vi "Lab Panel V4.83.vi"() -> ()   [LabVIEW 2013] (continued)
                  tunnel: w3955 -> [_ w3965]
                  frame False {
                  }
                  frame True {
                    n2340 = local read "TEMP START LAB03-1"() -> (w3971:cluster{"TL":dbl, "TN":dbl})
                    n2341 = local read "FAIL LAB03-1"() -> (w3962:cluster{"LO":dbl, "HI":dbl})
                    n2342 = local read "TDMS LAB03-1"() -> (w3970:refnum<k34>)
                    n2343 = local read "SET LAB03-1"() -> (w3967:T5)
                    n2344 = local read "DISP LAB03-1"() -> (w3968:T4)
                    n2345 = local read "SIG LAB03-1"() -> (w3972:T2)
                    n2346 = local read "RESULT LAB03-1"() -> (w3959:bool)
                    n2347 = Bundle("FAIL LAB03-1"=w3962, "SIG LAB03-1"=w3972, "TEMP START LAB03-1"=w3971, "DISP LAB03-1"=w3968, "SET LAB03-1"=w3967, "TDMS LAB03-1"=w3970) -> (w3957:T32)  [unwired: 1 in]
                    n2348 = call "sub vi - cycle&temp fail v6.vi"("Amps Lo?"=w3969, "Input Cluster"=w3957, "SELECT"=w3966, "Amps Hi?"=w3965, "Result In"=w3959) -> ("(FAIL) out"=w3961:cluster{"FAIL LO":dbl, "FAIL HI":dbl}, "(DISP) out"=w3964:T4, "T-RISE"=w3958:cluster{"T-RISE (L)":dbl, "T-RISE (N)":dbl}, "Result Out"=w3960:bool, "file error"=w3963:errorcluster)  [unwired: 10 in]
                    n2349 = local write "TEMP RISE LAB03-1"(w3958) -> ()
                    n2350 = local write "FAIL LAB03-1"(w3961) -> ()
                    n2351 = local write "DISP LAB03-1"(w3964) -> ()
                    n2352 = local write "RESULT LAB03-1"(w3960) -> ()
                    n2353 = local write "data file error"(w3963) -> ()
                  }
                }
              }
              frame #5 {
                # "LAB03-2"
                n2354 = case shown="True" w3974 {
                  tunnel: w3976 -> [_ w3989]
                  tunnel: w3973 -> [_ w3986]
                  tunnel: w3975 -> [_ w3985]
                  frame False {
                  }
                  frame True {
                    n2355 = local read "TEMP START LAB03-2"() -> (w3991:cluster{"TL":dbl, "TN":dbl})
                    n2356 = local read "FAIL LAB03-2"() -> (w3982:cluster{"LO":dbl, "HI":dbl})
                    n2357 = local read "TDMS LAB03-2"() -> (w3990:refnum<k34>)
                    n2358 = local read "SET LAB03-2"() -> (w3987:T5)
                    n2359 = local read "DISP LAB03-2"() -> (w3988:T4)
                    n2360 = local read "RESULT LAB03-2"() -> (w3979:bool)
                    n2361 = local read "SIG LAB03-2"() -> (w3992:T2)
                    n2362 = Bundle("FAIL LAB03-2"=w3982, "SIG LAB03-2"=w3992, "TEMP START LAB03-2"=w3991, "DISP LAB03-2"=w3988, "SET LAB03-2"=w3987, "TDMS LAB03-2"=w3990) -> (w3977:T33)  [unwired: 1 in]
                    n2363 = call "sub vi - cycle&temp fail v6.vi"("Amps Lo?"=w3989, "Input Cluster"=w3977, "SELECT"=w3986, "Amps Hi?"=w3985, "Result In"=w3979) -> ("(FAIL) out"=w3981:cluster{"FAIL LO":dbl, "FAIL HI":dbl}, "(DISP) out"=w3984:T4, "T-RISE"=w3978:cluster{"T-RISE (L)":dbl, "T-RISE (N)":dbl}, "Result Out"=w3980:bool, "file error"=w3983:errorcluster)  [unwired: 10 in]
                    n2364 = local write "FAIL LAB03-2"(w3981) -> ()
                    n2365 = local write "TEMP RISE LAB03-2"(w3978) -> ()
                    n2366 = local write "DISP LAB03-2"(w3984) -> ()
                    n2367 = local write "RESULT LAB03-2"(w3980) -> ()
                    n2368 = local write "data file error"(w3983) -> ()
                  }
                }
              }
              frame #6 {
                # "LAB04-1"
                n2369 = case shown="True" w3994 {
                  tunnel: w3996 -> [_ w4009]
                  tunnel: w3993 -> [_ w4006]
                  tunnel: w3995 -> [_ w4005]
                  frame False {
                  }
                  frame True {
                    n2370 = local read "TEMP START LAB04-1"() -> (w4011:cluster{"TL":dbl, "TN":dbl})
                    n2371 = local read "FAIL LAB04-1"() -> (w4002:cluster{"LO":dbl, "HI":dbl})
                    n2372 = local read "TDMS LAB04-1"() -> (w4010:refnum<k34>)
                    n2373 = local read "SET LAB04-1"() -> (w4007:T5)
                    n2374 = local read "DISP LAB04-1"() -> (w4008:T4)
                    n2375 = local read "SIG LAB04-1"() -> (w4012:T2)
                    n2376 = local read "RESULT LAB04-1"() -> (w3999:bool)
                    n2377 = Bundle("FAIL LAB04-1"=w4002, "SIG LAB04-1"=w4012, "TEMP START LAB04-1"=w4011, "DISP LAB04-1"=w4008, "SET LAB04-1"=w4007, "TDMS LAB04-1"=w4010) -> (w3997:T34)  [unwired: 1 in]
                    n2378 = call "sub vi - cycle&temp fail v6.vi"("Amps Lo?"=w4009, "Input Cluster"=w3997, "SELECT"=w4006, "Amps Hi?"=w4005, "Result In"=w3999) -> ("(FAIL) out"=w4001:cluster{"FAIL LO":dbl, "FAIL HI":dbl}, "(DISP) out"=w4004:T4, "T-RISE"=w3998:cluster{"T-RISE (L)":dbl, "T-RISE (N)":dbl}, "Result Out"=w4000:bool, "file error"=w4003:errorcluster)  [unwired: 10 in]
                    n2379 = local write "TEMP RISE LAB04-1"(w3998) -> ()
                    n2380 = local write "FAIL LAB04-1"(w4001) -> ()
                    n2381 = local write "DISP LAB04-1"(w4004) -> ()
                    n2382 = local write "RESULT LAB04-1"(w4000) -> ()
                    n2383 = local write "data file error"(w4003) -> ()
                  }
                }
              }
              frame #7 {
                # "LAB04-2"
                n2384 = case shown="True" w4014 {
                  tunnel: w4016 -> [_ w4029]
                  tunnel: w4013 -> [_ w4026]
                  tunnel: w4015 -> [_ w4025]
                  frame False {
                  }
                  frame True {
                    n2385 = local read "TEMP START LAB04-2"() -> (w4031:cluster{"TL":dbl, "TN":dbl})
                    n2386 = local read "FAIL LAB04-2"() -> (w4022:cluster{"LO":dbl, "HI":dbl})
                    n2387 = local read "TDMS LAB04-2"() -> (w4030:refnum<k34>)
                    n2388 = local read "SET LAB04-2"() -> (w4027:T5)
                    n2389 = local read "DISP LAB04-2"() -> (w4028:T4)
                    n2390 = local read "SIG LAB04-2"() -> (w4032:T2)
                    n2391 = local read "RESULT LAB04-2"() -> (w4019:bool)
                    n2392 = Bundle("FAIL LAB04-2"=w4022, "SIG LAB04-2"=w4032, "TEMP START LAB04-2"=w4031, "DISP LAB04-2"=w4028, "SET LAB04-2"=w4027, "TDMS LAB04-2"=w4030) -> (w4017:T35)  [unwired: 1 in]
                    n2393 = call "sub vi - cycle&temp fail v6.vi"("Amps Lo?"=w4029, "Input Cluster"=w4017, "SELECT"=w4026, "Amps Hi?"=w4025, "Result In"=w4019) -> ("(FAIL) out"=w4021:cluster{"FAIL LO":dbl, "FAIL HI":dbl}, "(DISP) out"=w4024:T4, "T-RISE"=w4018:cluster{"T-RISE (L)":dbl, "T-RISE (N)":dbl}, "Result Out"=w4020:bool, "file error"=w4023:errorcluster)  [unwired: 10 in]
                    n2394 = local write "TEMP RISE LAB04-2"(w4018) -> ()
                    n2395 = local write "FAIL LAB04-2"(w4021) -> ()
                    n2396 = local write "DISP LAB04-2"(w4024) -> ()
                    n2397 = local write "RESULT LAB04-2"(w4020) -> ()
                    n2398 = local write "data file error"(w4023) -> ()
                  }
                }
              }
              frame #8 {
                # "LAB05-1"
                n2399 = case shown="True" w4034 {
                  tunnel: w4036 -> [_ w4049]
                  tunnel: w4033 -> [_ w4046]
                  tunnel: w4035 -> [_ w4045]
                  frame False {
                  }
                  frame True {
                    n2400 = local read "TEMP START LAB05-1"() -> (w4051:cluster{"TL":dbl, "TN":dbl})
                    n2401 = local read "FAIL LAB05-1"() -> (w4042:cluster{"LO":dbl, "HI":dbl})
                    n2402 = local read "TDMS LAB05-1"() -> (w4050:refnum<k34>)
                    n2403 = local read "SET LAB05-1"() -> (w4047:T5)
                    n2404 = local read "DISP LAB05-1"() -> (w4048:T4)
                    n2405 = local read "SIG LAB05-1"() -> (w4052:T2)
                    n2406 = local read "RESULT LAB05-1"() -> (w4039:bool)
                    n2407 = Bundle("FAIL LAB05-1"=w4042, "SIG LAB05-1"=w4052, "TEMP START LAB05-1"=w4051, "DISP LAB05-1"=w4048, "SET LAB05-1"=w4047, "TDMS LAB05-1"=w4050) -> (w4037:T36)  [unwired: 1 in]
                    n2408 = call "sub vi - cycle&temp fail v6.vi"("Amps Lo?"=w4049, "Input Cluster"=w4037, "SELECT"=w4046, "Amps Hi?"=w4045, "Result In"=w4039) -> ("(FAIL) out"=w4041:cluster{"FAIL LO":dbl, "FAIL HI":dbl}, "(DISP) out"=w4044:T4, "T-RISE"=w4038:cluster{"T-RISE (L)":dbl, "T-RISE (N)":dbl}, "Result Out"=w4040:bool, "file error"=w4043:errorcluster)  [unwired: 10 in]
                    n2409 = local write "TEMP RISE LAB05-1"(w4038) -> ()
                    n2410 = local write "FAIL LAB05-1"(w4041) -> ()
                    n2411 = local write "DISP LAB05-1"(w4044) -> ()
                    n2412 = local write "RESULT LAB05-1"(w4040) -> ()
                    n2413 = local write "data file error"(w4043) -> ()
                  }
                }
              }
              frame #9 {
                # "LAB05-2"
                n2414 = case shown="True" w4054 {
                  tunnel: w4056 -> [_ w4069]
                  tunnel: w4053 -> [_ w4066]
                  tunnel: w4055 -> [_ w4065]
                  frame False {
                  }
                  frame True {
                    n2415 = local read "TEMP START LAB05-2"() -> (w4071:cluster{"TL":dbl, "TN":dbl})
                    n2416 = local read "FAIL LAB05-2"() -> (w4062:cluster{"LO":dbl, "HI":dbl})
                    n2417 = local read "TDMS LAB05-2"() -> (w4070:refnum<k34>)
                    n2418 = local read "SET LAB05-2"() -> (w4067:T5)
                    n2419 = local read "DISP LAB05-2"() -> (w4068:T4)
                    n2420 = local read "SIG LAB05-2"() -> (w4072:T2)
                    n2421 = local read "RESULT LAB05-2"() -> (w4059:bool)
                    n2422 = Bundle("FAIL LAB05-2"=w4062, "SIG LAB05-2"=w4072, "TEMP START LAB05-2"=w4071, "DISP LAB05-2"=w4068, "SET LAB05-2"=w4067, "TDMS LAB05-2"=w4070) -> (w4057:T37)  [unwired: 1 in]
                    n2423 = call "sub vi - cycle&temp fail v6.vi"("Amps Lo?"=w4069, "Input Cluster"=w4057, "SELECT"=w4066, "Amps Hi?"=w4065, "Result In"=w4059) -> ("(FAIL) out"=w4061:cluster{"FAIL LO":dbl, "FAIL HI":dbl}, "(DISP) out"=w4064:T4, "T-RISE"=w4058:cluster{"T-RISE (L)":dbl, "T-RISE (N)":dbl}, "Result Out"=w4060:bool, "file error"=w4063:errorcluster)  [unwired: 10 in]
                    n2424 = local write "TEMP RISE LAB05-2"(w4058) -> ()
                    n2425 = local write "FAIL LAB05-2"(w4061) -> ()
                    n2426 = local write "DISP LAB05-2"(w4064) -> ()
                    n2427 = local write "RESULT LAB05-2"(w4060) -> ()
                    n2428 = local write "data file error"(w4063) -> ()
                  }
                }
              }
            }
          }
          frame #15 {
            # "run calibration routine"
            n2429 = local read "CALIBRATE"() -> (w4073:bool)
            n2430 = case shown="True" w4073 {
              frame False {
              }
              frame True {
                n2431 = stacked-sequence {
                  seq-local: [w4074 _ _] -> [_ w4076 _]
                  frame #0 {
                    n2432 = call "CALIBRATION PASSWORD"() -> ("PASSWORD"=w4074:string)  [unwired: 17 in, 2 out]
                  }
                  frame #1 {
                    n2433 = Equal?(x=w4076, y="7777") -> (x = y?=w4075:bool)
                    n2434 = case shown="True" w4075 {
                      frame False {
                      }
                      frame True {
                        n2435 = stacked-sequence {
                          frame #0 {
                            n2436 = call "sub vi - calibration v1.vi"() -> ()  [unwired: 12 in]
                          }
                          frame #1 {
                            n2437 = call "sub vi - get calibration values v1.vi"() -> ("LAB01 (CAL)"=w4082:T9, "LAB02 (CAL)"=w4081:T10, "LAB03 (CAL)"=w4080:T9, "LAB04 (CAL)"=w4079:T9, "calibration file error out"=w4083:errorcluster, "LAB05 (CAL)"=w4078:T9)  [unwired: 10 in]
                            n2438 = local write "calibration file error out"(w4083) -> ()
                            n2439 = local write "CAL LAB04"(w4079) -> ()
                            n2440 = local write "CAL LAB05"(w4078) -> ()
                            n2441 = local write "CAL LAB01"(w4082) -> ()
                            n2442 = local write "CAL LAB02"(w4081) -> ()
                            n2443 = local write "CAL LAB03"(w4080) -> ()
                          }
                        }
                      }
                    }
                  }
                  frame #2 {
                    n2444 = local write "CALIBRATE"(FALSE) -> ()
                  }
                }
              }
            }
          }
          frame #16 {
            # "save certain settings to file"
            n2445 = String To Path(string="c:\\crabtree\\Set Up\\") -> (path=w4086:path)
            n2446 = Build Path(base path=w4086, name or relative path="settings.bin") -> (appended path=w4088:path)
            n2447 = Build Path(base path=w4086, name or relative path="mail.bin") -> (appended path=w4085:path)
            n2448 = Create Folder(path (use dialog)=w4086) -> (error out=w4091:errorcluster)  [unwired: 2 in, 2 out]
            n2449 = call <vilib>:"Clear Errors.vi"("error in (no error)"=w4091) -> ()  [unwired: 6 in, 1 out]
            n2450 = stacked-sequence {
              seq-local: [w4101 _] -> [_ w4114]
              tunnel: w4088 -> [_ w4115]
              tunnel: w4085 -> [_ w4113]
              frame #0 {
                n2451 = local read "C drive data root dir"() -> (w4100:path)
                n2452 = local read "Select COM port"() -> (w4097:refnum<visa-resource-name>)
                n2453 = local read "Network Directory"() -> (w4106:path)
                n2454 = local read "SET LAB05-2"() -> (w4105:T5)
                n2455 = local read "SET LAB05-1"() -> (w4104:T5)
                n2456 = local read "SET LAB04-2"() -> (w4103:T5)
                n2457 = local read "SET LAB03-2"() -> (w4107:T5)
                n2458 = local read "SET LAB04-1"() -> (w4102:T5)
                n2459 = local read "SET LAB03-1"() -> (w4108:T5)
                n2460 = local read "SET LAB02-2"() -> (w4109:T5)
                n2461 = local read "SET LAB02-1"() -> (w4110:T5)
                n2462 = local read "Temp Delay Lps"() -> (w4096:dbl)
                n2463 = local read "SET LAB01-2"() -> (w4111:T5)
                n2464 = local read "Temp Test Cal"() -> (w4093:dbl)
                n2465 = local read "SET LAB01-1"() -> (w4112:T5)
                n2466 = local read "Set Temp Lps"() -> (w4092:dbl)
                n2467 = local read "Temp Value"() -> (w4095:dbl)
                n2468 = local read "Fail Loops"() -> (w4094:dbl)
                n2469 = local read "RATE (Hz)"() -> (w4099:dbl)
                n2470 = local read "SAMPLES"() -> (w4098:dbl)
                n2471 = Bundle("SET LAB01-1"=w4112, "SET LAB01-2"=w4111, "SET LAB02-1"=w4110, "SET LAB02-2"=w4109, "SET LAB03-1"=w4108, "SET LAB03-2"=w4107, "SET LAB04-1"=w4102, "SET LAB04-2"=w4103, "SET LAB05-1"=w4104, "SET LAB05-2"=w4105, "Network Directory"=w4106, "C drive data root dir"=w4100, "RATE (Hz)"=w4099, "SAMPLES"=w4098, "Select COM port"=w4097, "Temp Delay Lps"=w4096, "Temp Value"=w4095, "Fail Loops"=w4094, "Temp Test Cal"=w4093, "Set Temp Lps"=w4092) -> (w4101:T20)  [unwired: 1 in]
              }
              frame #1 {
                n2472 = event shown="[1] \"SET LAB01-1\", \"SET LAB01-2\", \"SET LAB02-1\", \"SET LAB02-2\", \"SET LAB03-1\", \"SET LAB03-2\", \"SET LAB04-1\", \"SET LAB04-2\", \"SET LAB05-1\", \"SET LAB05-2\", \"Network Directory\", \"C drive data root dir\", \"RATE (Hz)\", \"SAMPLES\", \"Select COM port\", \"Temp Delay Lps\", \"Temp Value\", \"Fail Loops\", \"Temp Test Cal\", \"Set Temp Lps\": Value Change" {
                  selector: _ -> [_ _ _]
                  dyn-events: _ -> [_ _ _]
                  timeout: 10.0 -> [_ _ _]
                  tunnel: w4115 -> [_ w4117 _]
                  tunnel: w4114 -> [_ w4118 _]
                  tunnel: w4113 -> [_ _ w4129]
                  event Timeout {
                    n2473 = event-data() -> ()  [unwired: 1 in, 3 out]
                  }
                  event "SET LAB01-1", "SET LAB01-2", "SET LAB02-1", "SET LAB02-2", "SET LAB03-1", "SET LAB03-2", "SET LAB04-1", "SET LAB04-2", "SET LAB05-1", "SET LAB05-2", "Network Directory", "C drive data root dir", "RATE (Hz)", "SAMPLES", "Select COM port", "Temp Delay Lps", "Temp Value", "Fail Loops", "Temp Test Cal", "Set Temp Lps": Value Change {
                    n2474 = event-data() -> ()  [unwired: 1 in, 6 out]
                    n2475 = Open/Create/Replace File(file path (use dialog)=w4117, operation (0:open)=T19."replace or create") -> (refnum out=w4123:refnum<file>, error out=w4122:errorcluster)  [unwired: 4 in, 1 out]
                    n2476 = Write to Binary File(file (use dialog)=w4123, data=w4118, error in=w4122) -> (refnum out=w4121:refnum<file>, error out=w4120:errorcluster)  [unwired: 3 in, 1 out]
                    n2477 = Close File(refnum=w4121, error in=w4120) -> (error out=w4119:errorcluster)  [unwired: 1 out]
                    n2478 = local write "data file error"(w4119) -> ()
                  }
                  event "MAIL SETTINGS.OUT SERVER ADDRESS", "MAIL SETTINGS.FROM ACCOUNT", "MAIL SETTINGS.USER NAME", "MAIL SETTINGS.PASSWORD", "Auto Mail Send", "TO (string):": Value Change {
                    n2479 = event-data() -> ()  [unwired: 1 in, 6 out]
                    n2480 = local read "MAIL SETTINGS"() -> (w4128:T6)
                    n2481 = local read "Auto Mail Send"() -> (w4126:bool)
                    n2482 = local read "TO (string):"() -> (w4125:string)
                    n2483 = Open/Create/Replace File(file path (use dialog)=w4129, operation (0:open)=T19."replace or create") -> (refnum out=w4134:refnum<file>, error out=w4133:errorcluster)  [unwired: 4 in, 1 out]
                    n2484 = Bundle("MAIL SETTINGS"=w4128, "Auto Mail Send"=w4126, "TO (string):"=w4125) -> (w4127:T38)  [unwired: 1 in]
                    n2485 = Write to Binary File(file (use dialog)=w4134, data=w4127, error in=w4133) -> (refnum out=w4132:refnum<file>, error out=w4131:errorcluster)  [unwired: 3 in, 1 out]
                    n2486 = Close File(refnum=w4132, error in=w4131) -> (error out=w4130:errorcluster)  [unwired: 1 out]
                    n2487 = local write "data file error"(w4130) -> ()
                  }
                }
              }
            }
          }
          frame #17 {
            # "mail control"
            n2488 = local read "MAIL SETTINGS"() -> (w4151:T6)
            n2489 = local read "Auto Mail Send"() -> (w4137:bool)
            n2490 = Unbundle(w4151) -> ("OUT SERVER ADDRESS"=w4150:string, "FROM ACCOUNT"=w4149:string, "TEST MAIL"=w4148:bool)  [unwired: 4 out]
            n2491 = stacked-sequence {
              tunnel: "TO (string):" -> [_ w4190]
              tunnel: w4151 -> [w4156 w4189]
              tunnel: w4150 -> [w4155 w4188]
              tunnel: w4149 -> [w4154 w4187]
              tunnel: w4148 -> [w4153 _]
              tunnel: w4137 -> [_ w4186]
              tunnel: w4147 -> [_ w4185]
              tunnel: w4146 -> [_ w4184]
              tunnel: w4145 -> [_ w4183]
              tunnel: w4144 -> [_ w4182]
              tunnel: w4143 -> [_ w4181]
              tunnel: w4142 -> [_ w4180]
              tunnel: w4141 -> [_ w4179]
              tunnel: w4140 -> [_ w4178]
              tunnel: w4139 -> [_ w4177]
              tunnel: w4138 -> [_ w4176]
              tunnel: "TO (string):" -> [w4152 _]
              frame #0 {
                # "mail test"
                n2492 = case shown="True" w4153 {
                  tunnel: w4156 -> [_ w4160]
                  tunnel: w4152 -> [_ w4159]
                  tunnel: w4155 -> [_ w4158]
                  tunnel: w4154 -> [_ w4157]
                  frame False {
                  }
                  frame True {
                    n2493 = stacked-sequence {
                      seq-local: [_ _ w4170 _] -> [_ _ _ w4171]
                      tunnel: w4160 -> [w4163 _ _ w4175]
                      tunnel: w4159 -> [_ _ w4168 _]
                      tunnel: w4158 -> [_ _ w4166 _]
                      tunnel: w4157 -> [_ _ w4167 _]
                      frame #0 {
                        n2494 = Bundle(cluster=w4163, "TEST MAIL STATUS"="TEST START") -> (w4161:T6)  [unwired: 6 in]
                        n2495 = local write "MAIL SETTINGS"(w4161) -> ()
                      }
                      frame #1 {
                        n2496 = Wait (ms)(milliseconds to wait=500) -> ()  [unwired: 1 out]
                      }
                      frame #2 {
                        n2497 = call "sub vi - send mail with attach v5.vi"("TO:"=w4168, "subject"="MAIL TEST FROM LAB PANEL", "from"=w4167, "out going server"=w4166, "message"="TEST MESSAGE") -> ("error out"=w4170:errorcluster)  [unwired: 10 in]
                      }
                      frame #3 {
                        n2498 = Bundle(cluster=w4175, "TEST MAIL"=FALSE, "TEST MAIL STATUS"="TEST END", "mail error"=w4171) -> (w4173:T6)  [unwired: 4 in]
                        n2499 = local write "MAIL SETTINGS"(w4173) -> ()
                      }
                    }
                  }
                }
              }
              frame #1 {
                # "mail report"
                n2500 = stacked-sequence {
                  seq-local: [_ w4255 _ _] -> [_ _ _ w4423]
                  seq-local: [_ _ w4336 _] -> [_ _ _ w4413]
                  seq-local: [w4200 _ _ _] -> [_ w4249 _ _]
                  seq-local: [w4199 _ _ _] -> [_ w4248 _ _]
                  seq-local: [w4197 _ _ _] -> [_ w4246 _ _]
                  seq-local: [w4198 _ _ _] -> [_ w4247 _ _]
                  seq-local: [w4196 _ _ _] -> [_ w4245 _ _]
                  seq-local: [w4195 _ _ _] -> [_ w4240 _ _]
                  seq-local: [w4194 _ _ _] -> [_ w4241 _ _]
                  seq-local: [w4193 _ _ _] -> [_ w4242 _ _]
                  seq-local: [w4192 _ _ _] -> [_ w4243 _ _]
                  seq-local: [w4191 _ _ _] -> [_ w4244 _ _]
                  tunnel: w4190 -> [_ _ _ w4424]
                  tunnel: w4189 -> [_ _ _ w4407]
                  tunnel: w4188 -> [_ _ _ w4421]
                  tunnel: w4187 -> [_ _ _ w4420]
                  tunnel: w4186 -> [w4231 _ _ w4415]
                  tunnel: w4185 -> [_ _ w4366 _]
                  tunnel: w4184 -> [_ _ w4363 _]
                  tunnel: w4183 -> [_ _ w4362 _]
                  tunnel: w4182 -> [_ _ w4361 _]
                  tunnel: w4181 -> [_ _ w4360 _]
                  tunnel: w4180 -> [_ _ w4359 _]
                  tunnel: w4179 -> [_ _ w4358 _]
                  tunnel: w4178 -> [_ _ w4357 _]
                  tunnel: w4177 -> [_ _ w4356 _]
                  tunnel: w4176 -> [_ _ w4355 _]
                  frame #0 {
                    n2501 = case shown="False" w4231 {
                      frame False {
                        n2502 = local write "mail control"("") -> ()
                      }
                      frame True {
                      }
                    }
                    n2503 = local read "SET LAB01-1"() -> (w4230:T5)
                    n2504 = local read "SET LAB01-2"() -> (w4229:T5)
                    n2505 = local read "SET LAB02-1"() -> (w4228:T5)
                    n2506 = local read "SET LAB02-2"() -> (w4227:T5)
                    n2507 = local read "SET LAB03-1"() -> (w4226:T5)
                    n2508 = local read "SET LAB04-1"() -> (w4224:T5)
                    n2509 = local read "SET LAB05-1"() -> (w4222:T5)
                    n2510 = local read "SET LAB03-2"() -> (w4225:T5)
                    n2511 = local read "SET LAB04-2"() -> (w4223:T5)
                    n2512 = local read "SET LAB05-2"() -> (w4221:T5)
                    n2513 = Unbundle(w4226) -> ("DESCRIPTION"=w4206:string)  [unwired: 4 out]
                    n2514 = Unbundle(w4225) -> ("DESCRIPTION"=w4205:string)  [unwired: 4 out]
                    n2515 = Unbundle(w4224) -> ("DESCRIPTION"=w4204:string)  [unwired: 4 out]
                    n2516 = Unbundle(w4221) -> ("DESCRIPTION"=w4201:string)  [unwired: 4 out]
                    n2517 = Unbundle(w4227) -> ("DESCRIPTION"=w4207:string)  [unwired: 4 out]
                    n2518 = Unbundle(w4223) -> ("DESCRIPTION"=w4203:string)  [unwired: 4 out]
                    n2519 = Unbundle(w4230) -> ("DESCRIPTION"=w4219:string)  [unwired: 4 out]
                    n2520 = Unbundle(w4228) -> ("DESCRIPTION"=w4208:string)  [unwired: 4 out]
                    n2521 = Unbundle(w4222) -> ("DESCRIPTION"=w4202:string)  [unwired: 4 out]
                    n2522 = Unbundle(w4229) -> ("DESCRIPTION"=w4209:string)  [unwired: 4 out]
                    n2523 = Concatenate Strings("[LAB05-2/", w4201) -> (w4191:string)
                    n2524 = Concatenate Strings("[LAB05-1/", w4202) -> (w4192:string)
                    n2525 = Concatenate Strings("[LAB04-2/", w4203) -> (w4193:string)
                    n2526 = Concatenate Strings("[LAB03-2/", w4205) -> (w4195:string)
                    n2527 = Concatenate Strings("[LAB04-1/", w4204) -> (w4194:string)
                    n2528 = Concatenate Strings("[LAB03-1/", w4206) -> (w4196:string)
                    n2529 = Concatenate Strings("[LAB01-2/", w4209) -> (w4199:string)
                    n2530 = Concatenate Strings("[LAB02-2/", w4207) -> (w4197:string)
                    n2531 = Concatenate Strings("[LAB01-1/", w4219) -> (w4200:string)
                    n2532 = Concatenate Strings("[LAB02-1/", w4208) -> (w4198:string)
                  }
                  frame #1 {
                    w4253 = "/"
                    w4254 = 2.0
                    n2533 = local read "DISP LAB01-2"() -> (w4334:T4)
                    n2534 = local read "DISP LAB01-1"() -> (w4335:T4)
                    n2535 = local read "DISP LAB02-1"() -> (w4333:T4)
                    n2536 = local read "DISP LAB03-2"() -> (w4330:T4)
                    n2537 = local read "DISP LAB02-2"() -> (w4332:T4)
                    n2538 = local read "DISP LAB03-1"() -> (w4331:T4)
                    n2539 = local read "DISP LAB04-2"() -> (w4328:T4)
                    n2540 = local read "DISP LAB04-1"() -> (w4329:T4)
                    n2541 = local read "DISP LAB05-1"() -> (w4327:T4)
                    n2542 = local read "DISP LAB05-2"() -> (w4326:T4)
                    n2543 = Unbundle(w4334) -> ("CYCLE"=w4318:dbl, "MINS"=w4317:dbl, "STATUS"=w4314:string)
                    n2544 = Unbundle(w4335) -> ("CYCLE"=w4323:dbl, "MINS"=w4322:dbl, "STATUS"=w4319:string)
                    n2545 = Unbundle(w4333) -> ("CYCLE"=w4311:dbl, "MINS"=w4310:dbl, "STATUS"=w4309:string)
                    n2546 = Unbundle(w4330) -> ("CYCLE"=w4298:dbl, "MINS"=w4297:dbl, "STATUS"=w4294:string)
                    n2547 = Unbundle(w4331) -> ("CYCLE"=w4303:dbl, "MINS"=w4302:dbl, "STATUS"=w4299:string)
                    n2548 = Unbundle(w4332) -> ("CYCLE"=w4308:dbl, "MINS"=w4307:dbl, "STATUS"=w4304:string)
                    n2549 = Unbundle(w4329) -> ("CYCLE"=w4293:dbl, "MINS"=w4292:dbl, "STATUS"=w4289:string)
                    n2550 = Unbundle(w4328) -> ("CYCLE"=w4288:dbl, "MINS"=w4287:dbl, "STATUS"=w4284:string)
                    n2551 = Unbundle(w4327) -> ("CYCLE"=w4283:dbl, "MINS"=w4282:dbl, "STATUS"=w4279:string)
                    n2552 = Unbundle(w4326) -> ("CYCLE"=w4325:dbl, "MINS"=w4324:dbl, "STATUS"=w4276:string)
                    n2553 = Number To Decimal String(number=w4311) -> (decimal integer string=w4313:string)  [unwired: 1 in]
                    n2554 = Number To Decimal String(number=w4308) -> (decimal integer string=w4306:string)  [unwired: 1 in]
                    n2555 = Number To Decimal String(number=w4303) -> (decimal integer string=w4301:string)  [unwired: 1 in]
                    n2556 = Number To Decimal String(number=w4318) -> (decimal integer string=w4316:string)  [unwired: 1 in]
                    n2557 = Number To Decimal String(number=w4298) -> (decimal integer string=w4296:string)  [unwired: 1 in]
                    n2558 = Number To Decimal String(number=w4323) -> (decimal integer string=w4321:string)  [unwired: 1 in]
                    n2559 = Number To Decimal String(number=w4325) -> (decimal integer string=w4278:string)  [unwired: 1 in]
                    n2560 = Number To Decimal String(number=w4293) -> (decimal integer string=w4291:string)  [unwired: 1 in]
                    n2561 = Number To Decimal String(number=w4288) -> (decimal integer string=w4286:string)  [unwired: 1 in]
                    n2562 = Number To Decimal String(number=w4283) -> (decimal integer string=w4281:string)  [unwired: 1 in]
                    n2563 = Number To Fractional String(number=w4310, precision (6)=w4254) -> (F-format string=w4312:string)  [unwired: 2 in]
                    n2564 = Number To Fractional String(number=w4297, precision (6)=w4254) -> (F-format string=w4295:string)  [unwired: 2 in]
                    n2565 = Number To Fractional String(number=w4307, precision (6)=w4254) -> (F-format string=w4305:string)  [unwired: 2 in]
                    n2566 = Number To Fractional String(number=w4302, precision (6)=w4254) -> (F-format string=w4300:string)  [unwired: 2 in]
                    n2567 = Number To Fractional String(number=w4287, precision (6)=w4254) -> (F-format string=w4285:string)  [unwired: 2 in]
                    n2568 = Number To Fractional String(number=w4292, precision (6)=w4254) -> (F-format string=w4290:string)  [unwired: 2 in]
                    n2569 = Number To Fractional String(number=w4317, precision (6)=w4254) -> (F-format string=w4315:string)  [unwired: 2 in]
                    n2570 = Number To Fractional String(number=w4282, precision (6)=w4254) -> (F-format string=w4280:string)  [unwired: 2 in]
                    n2571 = Number To Fractional String(number=w4322, precision (6)=w4254) -> (F-format string=w4320:string)  [unwired: 2 in]
                    n2572 = Number To Fractional String(number=w4324, precision (6)=w4254) -> (F-format string=w4277:string)  [unwired: 2 in]
                    n2573 = Concatenate Strings(w4253, w4296, w4253, w4295, w4253, w4294) -> (w4270:string)
                    n2574 = Concatenate Strings(w4253, w4291, w4253, w4290, w4253, w4289) -> (w4269:string)
                    n2575 = Concatenate Strings(w4253, w4286, w4253, w4285, w4253, w4284) -> (w4268:string)
                    n2576 = Concatenate Strings(w4253, w4281, w4253, w4280, w4253, w4279) -> (w4267:string)
                    n2577 = Concatenate Strings(w4253, w4278, w4253, w4277, w4253, w4276) -> (w4266:string)
                    n2578 = Concatenate Strings(w4253, w4321, w4253, w4320, w4253, w4319) -> (w4275:string)
                    n2579 = Concatenate Strings(w4253, w4301, w4253, w4300, w4253, w4299) -> (w4271:string)
                    n2580 = Concatenate Strings(w4253, w4316, w4253, w4315, w4253, w4314) -> (w4274:string)
                    n2581 = Concatenate Strings(w4253, w4313, w4253, w4312, w4253, w4309) -> (w4273:string)
                    n2582 = Concatenate Strings(w4253, w4306, w4253, w4305, w4253, w4304) -> (w4272:string)
                    n2583 = Concatenate Strings("]", "\r") -> (w4250:string)
                    n2584 = Concatenate Strings(w4245, w4271, w4250) -> (w4261:string)
                    n2585 = Concatenate Strings(w4247, w4273, w4250) -> (w4263:string)
                    n2586 = Concatenate Strings(w4246, w4272, w4250) -> (w4262:string)
                    n2587 = Concatenate Strings(w4242, w4268, w4250) -> (w4258:string)
                    n2588 = Concatenate Strings(w4243, w4267, w4250) -> (w4259:string)
                    n2589 = Concatenate Strings(w4241, w4269, w4250) -> (w4257:string)
                    n2590 = Concatenate Strings(w4240, w4270, w4250) -> (w4256:string)
                    n2591 = Concatenate Strings(w4244, w4266, w4250) -> (w4260:string)
                    n2592 = Concatenate Strings(w4248, w4274, w4250) -> (w4264:string)
                    n2593 = Concatenate Strings(w4249, w4275, w4250) -> (w4265:string)
                    n2594 = Concatenate Strings(w4265, w4264, w4263, w4262, w4261, w4256, w4257, w4258, w4259, w4260) -> (w4233:string)
                    n2595 = Concatenate Strings("[PANEL/", "DESC/", "CYCLES/", "MINS/", "STATUS]", "\r", w4233) -> (w4255:string)
                    "MAIL REPORT" <- w4255
                  }
                  frame #2 {
                    w4364 = "END"
                    n2596 = local read "mail control"() -> (w4365:string)
                    n2597 = case shown="False" w4360 {
                      tunnel: w4365 -> [w4389 _]
                      tunnel: w4364 -> [w4388 _]
                      tunnel: [w4387 FALSE] -> w4350
                      frame False {
                        n2598 = Equal?(x=w4389, y=w4388) -> (x = y?=w4387:bool)
                      }
                      frame True {
                      }
                    }
                    n2599 = case shown="False" w4366 {
                      tunnel: w4365 -> [w4405 _]
                      tunnel: w4364 -> [w4404 _]
                      tunnel: [w4403 FALSE] -> w4354
                      frame False {
                        n2600 = Equal?(x=w4405, y=w4404) -> (x = y?=w4403:bool)
                      }
                      frame True {
                      }
                    }
                    n2601 = case shown="False" w4363 {
                      tunnel: w4365 -> [w4401 _]
                      tunnel: w4364 -> [w4400 _]
                      tunnel: [w4399 FALSE] -> w4353
                      frame False {
                        n2602 = Equal?(x=w4401, y=w4400) -> (x = y?=w4399:bool)
                      }
                      frame True {
                      }
                    }
                    n2603 = case shown="False" w4361 {
                      tunnel: w4365 -> [w4393 _]
                      tunnel: w4364 -> [w4392 _]
                      tunnel: [w4391 FALSE] -> w4351
                      frame False {
                        n2604 = Equal?(x=w4393, y=w4392) -> (x = y?=w4391:bool)
                      }
                      frame True {
                      }
                    }
                    n2605 = case shown="False" w4362 {
                      tunnel: w4365 -> [w4397 _]
                      tunnel: w4364 -> [w4396 _]
                      tunnel: [w4395 FALSE] -> w4352
                      frame False {
                        n2606 = Equal?(x=w4397, y=w4396) -> (x = y?=w4395:bool)
                      }
                      frame True {
                      }
                    }
                    n2607 = Or(x=w4352, y=w4351) -> (x .or. y?=w4343:bool)
                    n2608 = Or(x=w4354, y=w4353) -> (x .or. y?=w4344:bool)
                    n2609 = Or(x=w4344, y=w4343) -> (x .or. y?=w4339:bool)
                    n2610 = case shown="False" w4356 {
                      tunnel: w4365 -> [w4373 _]
                      tunnel: w4364 -> [w4372 _]
                      tunnel: [w4371 FALSE] -> w4345
                      frame False {
                        n2611 = Equal?(x=w4373, y=w4372) -> (x = y?=w4371:bool)
                      }
                      frame True {
                      }
                    }
                    n2612 = case shown="False" w4355 {
                      tunnel: w4365 -> [w4369 _]
                      tunnel: w4364 -> [w4368 _]
                      tunnel: [w4367 FALSE] -> w4349
                      frame False {
                        n2613 = Equal?(x=w4369, y=w4368) -> (x = y?=w4367:bool)
                      }
                      frame True {
                      }
                    }
                    n2614 = case shown="False" w4357 {
                      tunnel: w4365 -> [w4377 _]
                      tunnel: w4364 -> [w4376 _]
                      tunnel: [w4375 FALSE] -> w4346
                      frame False {
                        n2615 = Equal?(x=w4377, y=w4376) -> (x = y?=w4375:bool)
                      }
                      frame True {
                      }
                    }
                    n2616 = case shown="False" w4359 {
                      tunnel: w4365 -> [w4385 _]
                      tunnel: w4364 -> [w4384 _]
                      tunnel: [w4383 FALSE] -> w4348
                      frame False {
                        n2617 = Equal?(x=w4385, y=w4384) -> (x = y?=w4383:bool)
                      }
                      frame True {
                      }
                    }
                    n2618 = case shown="False" w4358 {
                      tunnel: w4365 -> [w4381 _]
                      tunnel: w4364 -> [w4380 _]
                      tunnel: [w4379 FALSE] -> w4347
                      frame False {
                        n2619 = Equal?(x=w4381, y=w4380) -> (x = y?=w4379:bool)
                      }
                      frame True {
                      }
                    }
                    n2620 = Or(x=w4348, y=w4347) -> (x .or. y?=w4342:bool)
                    n2621 = Or(x=w4346, y=w4345) -> (x .or. y?=w4341:bool)
                    n2622 = Or(x=w4349, y=w4350) -> (x .or. y?=w4337:bool)
                    n2623 = Or(x=w4342, y=w4341) -> (x .or. y?=w4340:bool)
                    n2624 = Or(x=w4339, y=w4340) -> (x .or. y?=w4338:bool)
                    n2625 = Or(x=w4338, y=w4337) -> (x .or. y?=w4336:bool)
                  }
                  frame #3 {
                    n2626 = local read "on loops"() -> (w4419:dbl)
                    n2627 = local read "jig cycle"() -> (w4416:dbl)
                    n2628 = local read "Send Mail Now"() -> (w4410:bool)
                    n2629 = Add(x=w4419, y=3.0) -> (x+y=w4417:dbl)
                    n2630 = Equal?(x=w4416, y=w4417) -> (x = y?=w4411:bool)
                    n2631 = And(x=w4411, y=w4410) -> (x .and. y?=w4409:bool)
                    n2632 = And(x=w4415, y=w4411) -> (x .and. y?=w4414:bool)
                    n2633 = And(x=w4414, y=w4413) -> (x .and. y?=w4412:bool)
                    n2634 = Or(x=w4412, y=w4409) -> (x .or. y?=w4408:bool)
                    n2635 = case shown="True" w4408 {
                      tunnel: w4424 -> [_ w4430]
                      tunnel: w4423 -> [_ w4429]
                      tunnel: "Lab Panel Test Status" -> [_ w4428]
                      tunnel: w4421 -> [_ w4427]
                      tunnel: w4420 -> [_ w4426]
                      tunnel: w4407 -> [_ w4425]
                      frame False {
                      }
                      frame True {
                        n2636 = stacked-sequence {
                          tunnel: w4430 -> [w4438 _]
                          tunnel: w4429 -> [w4437 _]
                          tunnel: w4428 -> [w4436 _]
                          tunnel: w4427 -> [w4435 _]
                          tunnel: w4426 -> [w4434 _]
                          tunnel: w4425 -> [w4433 _]
                          frame #0 {
                            n2637 = call "sub vi - send mail with attach v5.vi"("TO:"=w4438, "subject"=w4436, "from"=w4434, "out going server"=w4435, "message"=w4437) -> ("error out"=w4432:errorcluster)  [unwired: 10 in]
                            n2638 = Bundle(cluster=w4433, "mail error"=w4432) -> (w4431:T6)  [unwired: 6 in]
                            n2639 = local write "MAIL SETTINGS"(w4431) -> ()
                          }
                          frame #1 {
                            n2640 = local write "mail control"("") -> ()
                            n2641 = local write "Send Mail Now"(FALSE) -> ()
                          }
                        }
                      }
                    }
                  }
                }
              }
            }
          }
          frame #18 {
            # "save jig cycle values once all run switches are off"
            n2642 = stacked-sequence {
              tunnel: w4450 -> [_ w4479]
              tunnel: w4449 -> [_ w4478]
              tunnel: w4448 -> [_ w4477]
              tunnel: w4447 -> [_ w4476]
              tunnel: w4446 -> [_ w4475]
              tunnel: w4445 -> [_ w4474]
              tunnel: w4444 -> [_ w4473]
              tunnel: w4443 -> [_ w4472]
              tunnel: w4442 -> [_ w4471]
              tunnel: w4441 -> [_ w4470]
              frame #0 {
              }
              frame #1 {
                n2643 = Not(x=w4470) -> (.not. x?=w4453:bool)
                n2644 = Not(x=w4478) -> (.not. x?=w4468:bool)
                n2645 = Not(x=w4475) -> (.not. x?=w4463:bool)
                n2646 = Not(x=w4473) -> (.not. x?=w4459:bool)
                n2647 = Not(x=w4471) -> (.not. x?=w4455:bool)
                n2648 = Not(x=w4479) -> (.not. x?=w4469:bool)
                n2649 = Not(x=w4477) -> (.not. x?=w4467:bool)
                n2650 = Not(x=w4474) -> (.not. x?=w4461:bool)
                n2651 = Not(x=w4476) -> (.not. x?=w4465:bool)
                n2652 = Not(x=w4472) -> (.not. x?=w4457:bool)
                n2653 = local read "Save JC"() -> (w4481:bool)
                n2654 = And(x=w4469, y=w4468) -> (x .and. y?=w4466:bool)
                n2655 = And(x=w4466, y=w4467) -> (x .and. y?=w4464:bool)
                n2656 = And(x=w4464, y=w4465) -> (x .and. y?=w4462:bool)
                n2657 = And(x=w4462, y=w4463) -> (x .and. y?=w4460:bool)
                n2658 = And(x=w4460, y=w4461) -> (x .and. y?=w4458:bool)
                n2659 = And(x=w4458, y=w4459) -> (x .and. y?=w4456:bool)
                n2660 = And(x=w4456, y=w4457) -> (x .and. y?=w4454:bool)
                n2661 = And(x=w4454, y=w4455) -> (x .and. y?=w4452:bool)
                n2662 = And(x=w4452, y=w4453) -> (x .and. y?=w4451:bool)
                n2663 = And(x=w4451, y=w4481) -> (x .and. y?=w4480:bool)
                n2664 = case shown="True" w4480 {
                  tunnel: w4451 -> [w4482 _]
                  frame False {
                    n2665 = case shown="False" w4482 {
                      frame False {
                        n2666 = local write "Save JC"(TRUE) -> ()
                      }
                      frame True {
                      }
                    }
                  }
                  frame True {
                    n2667 = stacked-sequence {
                      frame #0 {
                        n2668 = String To Path(string="c:\\crabtree\\Jig Cycles\\") -> (path=w4494:path)
                        n2669 = Build Path(base path=w4494, name or relative path="jigcycles.bin") -> (appended path=w4492:path)
                        n2670 = Create Folder(path (use dialog)=w4494) -> (error out=w4496:errorcluster)  [unwired: 2 in, 2 out]
                        n2671 = local read "JIG RELAY CYCLES"() -> (w4486:T7)
                        n2672 = call <vilib>:"Clear Errors.vi"("error in (no error)"=w4496) -> ()  [unwired: 6 in, 1 out]
                        n2673 = local write "Save JC"(FALSE) -> ()
                        n2674 = Open/Create/Replace File(file path (use dialog)=w4492, operation (0:open)=T19."replace or create") -> (refnum out=w4490:refnum<file>, error out=w4491:errorcluster)  [unwired: 4 in, 1 out]
                        n2675 = Write to Binary File(file (use dialog)=w4490, data=w4486, error in=w4491) -> (refnum out=w4489:refnum<file>, error out=w4488:errorcluster)  [unwired: 3 in, 1 out]
                        n2676 = Close File(refnum=w4489, error in=w4488) -> (error out=w4487:errorcluster)  [unwired: 1 out]
                        n2677 = local write "data file error"(w4487) -> ()
                      }
                      frame #1 {
                        n2678 = local read "JIG RELAY CYCLES"() -> (w4519:T7)
                        n2679 = Unbundle By Name(w4519) -> ("LAB01-1"=w4514:dbl, "LAB01-2"=w4513:dbl, "LAB02-1"=w4511:dbl, "LAB02-2"=w4510:dbl, "LAB03-1"=w4508:dbl, "LAB03-2"=w4505:dbl, "LAB04-1"=w4504:dbl, "LAB04-2"=w4502:dbl, "LAB05-1"=w4500:dbl, "LAB05-2"=w4498:dbl)
                        n2680 = stacked-sequence {
                          tunnel: w4514 -> [w4522 _ _ _ _ _ _ _ _ _]
                          tunnel: 1000000 -> [w4525 w4535 w4545 w4555 w4565 w4575 w4585 w4595 w4605 w4615]
                          tunnel: [w4523 _ _ _ _ _ _ _ _ _] -> w4517
                          tunnel: "TEST STATION HAS REACHED 1 MILLION CYCLES, REPLACE  CONTROL RELAYS" -> [w4521 w4533 w4543 w4553 w4563 w4573 w4583 w4593 w4603 w4613]
                          tunnel: [_ w4532 _ _ _ _ _ _ _ _] -> w4515
                          tunnel: w4513 -> [_ w4531 _ _ _ _ _ _ _ _]
                          tunnel: [_ _ w4542 _ _ _ _ _ _ _] -> w4512
                          tunnel: w4511 -> [_ _ w4541 _ _ _ _ _ _ _]
                          tunnel: w4510 -> [_ _ _ w4552 _ _ _ _ _ _]
                          tunnel: [_ _ _ w4551 _ _ _ _ _ _] -> w4509
                          tunnel: w4508 -> [_ _ _ _ w4562 _ _ _ _ _]
                          tunnel: [_ _ _ _ w4561 _ _ _ _ _] -> w4507
                          tunnel: [_ _ _ _ _ w4572 _ _ _ _] -> w4506
                          tunnel: w4505 -> [_ _ _ _ _ w4571 _ _ _ _]
                          tunnel: w4504 -> [_ _ _ _ _ _ w4582 _ _ _]
                          tunnel: [_ _ _ _ _ _ w4581 _ _ _] -> w4503
                          tunnel: w4502 -> [_ _ _ _ _ _ _ w4592 _ _]
                          tunnel: [_ _ _ _ _ _ _ w4591 _ _] -> w4501
                          tunnel: w4500 -> [_ _ _ _ _ _ _ _ w4602 _]
                          tunnel: [_ _ _ _ _ _ _ _ w4601 _] -> w4499
                          tunnel: w4498 -> [_ _ _ _ _ _ _ _ _ w4612]
                          tunnel: [_ _ _ _ _ _ _ _ _ w4611] -> w4497
                          frame #0 {
                            n2681 = Greater?(x=w4522, y=w4525) -> (0:w4524:bool)
                            n2682 = case shown="True" w4524 {
                              tunnel: [w4526 0] -> w4523
                              tunnel: w4522 -> [w4526 _]
                              tunnel: w4521 -> [_ w4527]
                              frame False {
                              }
                              frame True {
                                n2683 = Concatenate Strings("LA01-1 ", w4527) -> (w4530:string)
                                n2684 = One Button Dialog(message=w4530) -> ()  [unwired: 1 in, 1 out]
                              }
                            }
                          }
                          frame #1 {
                            n2685 = Greater?(x=w4531, y=w4535) -> (0:w4534:bool)
                            n2686 = case shown="True" w4534 {
                              tunnel: [w4536 0] -> w4532
                              tunnel: w4531 -> [w4536 _]
                              tunnel: w4533 -> [_ w4537]
                              frame False {
                              }
                              frame True {
                                n2687 = Concatenate Strings("LA01-2 ", w4537) -> (w4540:string)
                                n2688 = One Button Dialog(message=w4540) -> ()  [unwired: 1 in, 1 out]
                              }
                            }
                          }
                          frame #2 {
                            n2689 = Greater?(x=w4541, y=w4545) -> (0:w4544:bool)
                            n2690 = case shown="True" w4544 {
                              tunnel: [w4546 0] -> w4542
                              tunnel: w4541 -> [w4546 _]
                              tunnel: w4543 -> [_ w4547]
                              frame False {
                              }
                              frame True {
                                n2691 = Concatenate Strings("LA02-1 ", w4547) -> (w4550:string)
                                n2692 = One Button Dialog(message=w4550) -> ()  [unwired: 1 in, 1 out]
                              }
                            }
                          }
                          frame #3 {
                            n2693 = Greater?(x=w4552, y=w4555) -> (0:w4554:bool)
                            n2694 = case shown="True" w4554 {
                              tunnel: [w4556 0] -> w4551
                              tunnel: w4552 -> [w4556 _]
                              tunnel: w4553 -> [_ w4557]
                              frame False {
                              }
                              frame True {
                                n2695 = Concatenate Strings("LA02-2 ", w4557) -> (w4560:string)
                                n2696 = One Button Dialog(message=w4560) -> ()  [unwired: 1 in, 1 out]
                              }
                            }
                          }
                          frame #4 {
                            n2697 = Greater?(x=w4562, y=w4565) -> (0:w4564:bool)
                            n2698 = case shown="True" w4564 {
                              tunnel: [w4566 0] -> w4561
